vi "Matches.vi"(8 "error in (no error)":errorcluster, 10 "Actual":variant, 11 "Is Same Type in":refnum<class "Is Same Type.lvclass">) -> (0 "error out":errorcluster, 2 "Result":bool, 3 "Is Same Type out":refnum<class "Is Same Type.lvclass">)   [LabVIEW 2017, in "Transparent Assertions.lvlib" / "Is Same Type.lvclass"]
doc: "Evaluates the constraint for <B>Actual</B>. Returns true if the constraint is met."
uses:
  Is Same Type.lvclass
  Is Same Type.lvclass/Is Same Type.ctl
  <vilib>/Utility/Data Type/NI_Data Type.lvlib
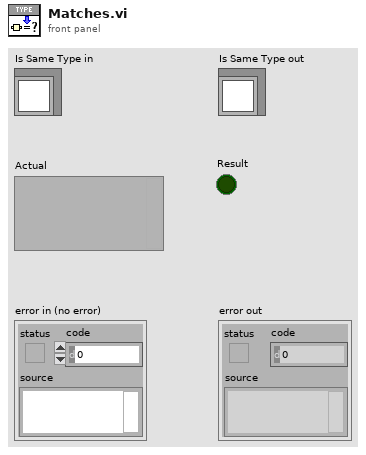
[diagram p1: front panel]
types:
  T1 = typedef "NI_Data Type.lvlib/Data Type.ctl" = enum8{"Invalid Type", "Void", "I8", "I16", "I32", "I64", "U8", "U16", "U32", "U64", "Single Float", "Double Float", "Extended Float", "Single Complex", "Double Complex", "Extended Complex", "Enum U8", "Enum U16", "Enum U32", "Enum U64", "Single Float With Unit", "Double Float With Unit", "Extended Float With Unit", "Single Complex with Unit", "Double Complex with Unit", "Extended Complex with Unit", "Boolean", "String", "Path", "Picture", "Tag", "Array", "Cluster", "Variant", "LV Variant", "Waveform", "Timestamp", "Digital Waveform", "Digital Data", "ExpressData", "Refnum", "External Data", "VI", "Poly VI", "LabVIEW Class Instance", "Fixed Point"}
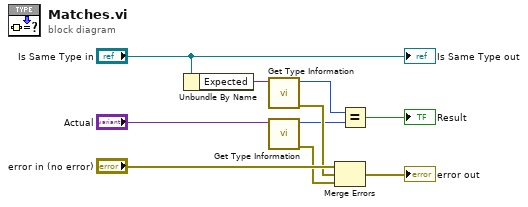
[diagram p0: block diagram]
diagram:
  n1 = Unbundle By Name("Is Same Type in") -> ("Expected"=w8:variant)
  n2 = call <vilib>:"Get Type Information.vi"("Variant"=w8) -> ("error out"=w6:errorcluster, "Type"=w2:T1)  [unwired: 6 in, 3 out]
  n3 = call <vilib>:"Get Type Information.vi"("Variant"="Actual") -> ("error out"=w5:errorcluster, "Type"=w3:T1)  [unwired: 6 in, 3 out]
  n4 = Merge Errors("error in (no error)", w6, w5) -> (→"error out":errorcluster)
  n5 = Equal?(x=w2, y=w3) -> (x = y?=→"Result":bool)
  "Is Same Type out" <- "Is Same Type in"
